vi "read from CE14(SubVI).vi"(8 "error in (no error)":errorcluster, 9 "Time out ms (1000)":u32=1000, 11 "COMport in":refnum<visa-resource-name>) -> (0 "error out":errorcluster, 1 "Time out":bool, 2 "received msg":string, 3 "COMport out":refnum<visa-resource-name>)   [LabVIEW 2018]
uses:
  CE14_eMIC.lvlib
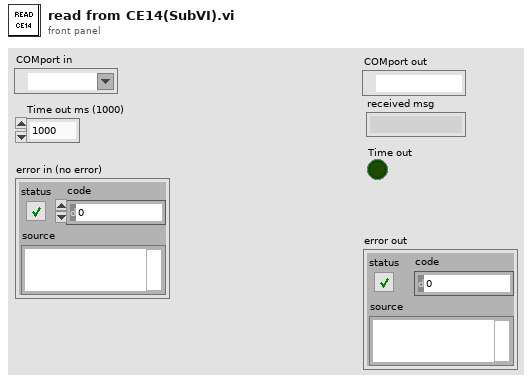
[diagram p1: front panel]
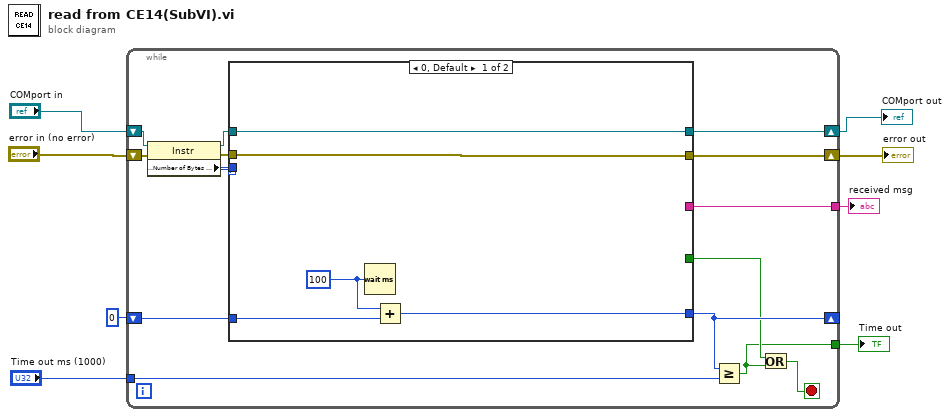
[diagram p0: block diagram]
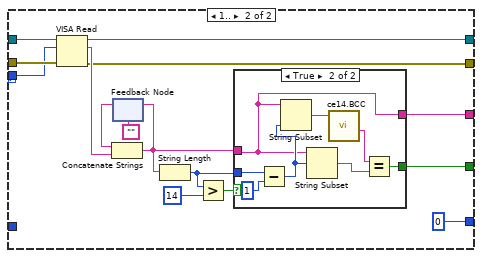
[diagram p2: hidden frame]
diagram:
  n1 = while {
    tunnel: "Time out ms (1000)" -> [w16]
    shift-right: [w17] -> _
    shift-left: u32 0 -> [w18]
    tunnel: [w13] -> w6
    tunnel: [w12] -> w1
    shift-right: [w11] -> w3
    shift-left: "COMport in" -> [w20]
    shift-right: [w10] -> w4
    shift-left: "error in (no error)" -> [w9]
    stop <- w14 stop-if-true
    n2 = property class="Instr"(reference=w20, error in=w9) -> (reference out=w21:refnum<visa-resource-name>, error out=w22:errorcluster, "Serial Settings:Number of Bytes at Serial Port"=w19:u32)
    n3 = case shown="0, Default" w19 {
      tunnel: w22 -> [w23 w42]
      tunnel: w21 -> [w24 w41]
      tunnel: w19 -> [_ w40]
      tunnel: w18 -> [w26 _]
      tunnel: [w25 u32 0] -> w17
      tunnel: [_ w31] -> w15
      tunnel: [_ w30] -> w12
      tunnel: [w24 w29] -> w11
      tunnel: [w23 w28] -> w10
      frame 0, Default {
        w27 = u32 100 ("milliseconds to wait")
        n4 = Wait (ms)(milliseconds to wait=w27) -> ()  [unwired: 1 out]
        n5 = Add(x=w27, y=w26) -> (x+y=w25:u32)
      }
      frame 1.. {
        n6 = VISA Read(VISA resource name=w41, byte count=w40, error in (no error)=w42) -> (VISA resource name out=w29:refnum<visa-resource-name>, read buffer=w38:string, error out=w28:errorcluster)  [unwired: 1 out]
        n7 = feedback #1("") -> (w37:string)
        n8 = Concatenate Strings(w37, w38) -> (w33:string)
        n9 = feedback-in #1(w33) -> ()
        n10 = String Length(string=w33) -> (length=w32:i32)
        n11 = Greater?(x=w32, y=14) -> (0:w34:bool)
        n12 = case shown="True" w34 {
          tunnel: w33 -> [w43 w44]
          tunnel: w32 -> [_ w51]
          tunnel: [_ w45] -> w31
          tunnel: [w43 w44] -> w30
          frame False {
          }
          frame True {
            n13 = Subtract(x=w51, y=1) -> (x-y=w48:i32)
            n14 = String Subset(string=w44, length (rest)=w48) -> (substring=w49:string)  [unwired: 1 in]
            n15 = String Subset(string=w44, offset (0)=w48) -> (substring=w46:string)  [unwired: 1 in]
            n16 = call "ce14.BCC.vi"("mess in"=w49) -> ("BCC"=w47:string)  [unwired: 8 in, 2 out]
            n17 = Equal?(x=w47, y=w46) -> (x = y?=w45:bool)
          }
        }
      }
    }
    n18 = Greater Or Equal?(x=w17, y=w16) -> (x >= y?=w13:bool)
    n19 = Or(x=w15, y=w13) -> (x .or. y?=w14:bool)
  }
  "Time out" <- w6
  "error out" <- w4
  "COMport out" <- w3
  "received msg" <- w1
